vi "Create From Variant (Boolean).vi"(8 "error in (no error)":errorcluster, 10 "Variant":variant, 11 "JSON Boolean in":refnum<class "JSON Value.lvclass">) -> (0 "error out":errorcluster, 3 "JSON Boolean out":refnum<class "JSON Value.lvclass">)   [LabVIEW 2016, in "JSON Value.lvclass"]
doc: "Creates a new JSON instance from the given Variant."
uses:
  JSON Helper/JSON Value.lvclass
  JSON Helper/JSON Value.lvclass/JSON Value.ctl
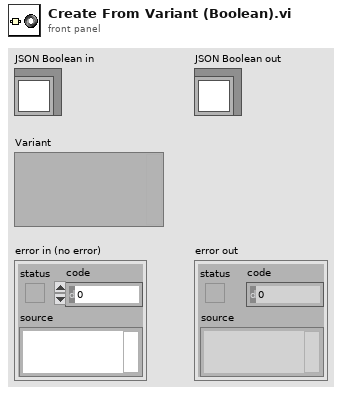
[diagram p1: front panel]
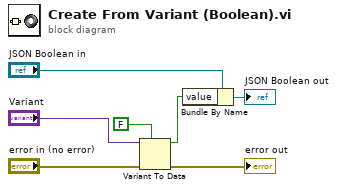
[diagram p0: block diagram]
diagram:
  n1 = Variant To Data(error in="error in (no error)", type=FALSE, Variant="Variant") -> (data=w4:bool, error out=→"error out":errorcluster)
  n2 = Bundle By Name(cluster="JSON Boolean in", "value"=w4) -> (→"JSON Boolean out":refnum<class "JSON Value.lvclass">)
